vi "get_additional_soft_limit_XYZ.vi"(8 "error in (no error)":errorcluster caption="错误输入（无错误）", 11 "MotorSystem 输入":refnum<class "MotorSystem.lvclass">) -> (0 "error out":errorcluster caption="错误输出", 2 "additional soft limit":T1(array[cluster]), 3 "MotorSystem 输出":refnum<class "MotorSystem.lvclass">)   [LabVIEW 2016, in "MotionControl.lvlib" / "MotorSystem.lvclass"]
uses:
  <userlib>/MotionControl/MotorSystem/MotorSystem.lvclass
  <userlib>/MotionControl/MotorSystem/MotorSystem.lvclass/MotorSystem.ctl
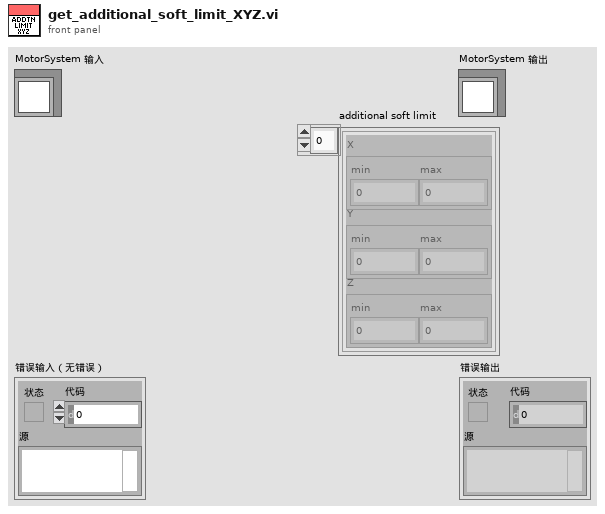
[diagram p1: front panel]
types:
  T1 = cluster{"X":cluster{"min":dbl, "max":dbl}, "Y":cluster{"min":dbl, "max":dbl}, "Z":cluster{"min":dbl, "max":dbl}}[]
  T2 = cluster{"array for a soft limit":cluster{"dim name":string, "soft limit":cluster{"min":dbl, "max":dbl}}[]}[]
  T3 = cluster{"dim name":string, "soft limit":cluster{"min":dbl, "max":dbl}}[]
  T4 = cluster{"[0]":cluster{"min":dbl, "max":dbl}, "[1]":cluster{"min":dbl, "max":dbl}, "[2]":cluster{"min":dbl, "max":dbl}}
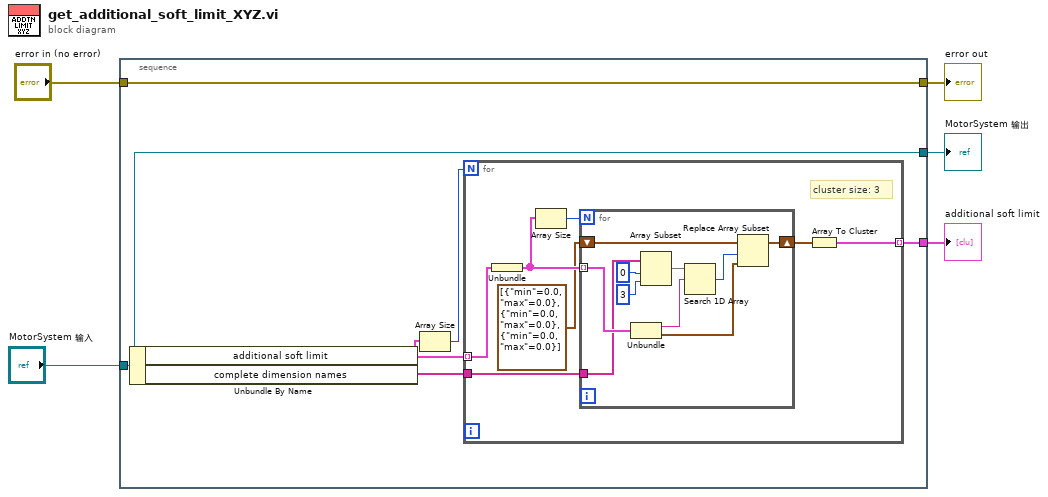
[diagram p0: block diagram]
diagram:
  n1 = stacked-sequence {
    tunnel: [w11] -> w5
    tunnel: [w10] -> w3
    tunnel: "MotorSystem 输入" -> [w10]
    tunnel: "error in (no error)" -> [w11]
    tunnel: [w6] -> w1
    frame #0 {
      n2 = Unbundle By Name(w10) -> ("additional soft limit"=w9:T2, "complete dimension names"=w7:string[])
      n3 = Array Size(array=w9) -> (size(s)=w8:i32)
      n4 = for {
        N: w8 -> [_]
        tunnel: w9 -> [w18] mode=indexing
        tunnel: w7 -> [w15]
        tunnel: [w12] -> w6 mode=indexing
        # "cluster size: 3"
        n5 = Unbundle(w18) -> ("array for a soft limit"=w17:T3)
        n6 = Array Size(array=w17) -> (size(s)=w16:i32)
        n7 = for {
          N: w16 -> [_]
          tunnel: w17 -> [w28] mode=indexing
          tunnel: w15 -> [w27]
          shift-right: [w19] -> w13
          shift-left: cluster{"min":dbl, "max":dbl}[] [{"min"=0.0, "max"=0.0}, {"min"=0.0, "max"=0.0}, {"min"=0.0, "max"=0.0}] -> [w22]
          n8 = Unbundle(w28) -> ("dim name"=w23:string, "soft limit"=w20:cluster{"min":dbl, "max":dbl})
          n9 = Array Subset(array=w27, index=0 ("索引"), length=3 ("长度")) -> (w24:string[])
          n10 = Search 1D Array(1D array=w24, element=w23) -> (index of element=w21:i32)  [unwired: 1 in]
          n11 = Replace Array Subset(array=w22, new element=w20, index=w21) -> (w19:cluster{"min":dbl, "max":dbl}[])
        }
        n12 = Array To Cluster(array=w13) -> (cluster=w12:T4)
      }
    }
  }
  "error out" <- w5
  "MotorSystem 输出" <- w3
  "additional soft limit" <- w1
